vi "temperature calling.vi"() -> ()   [LabVIEW 2018]
panel:
  in  "Boolean":bool
  out "Thermometer":dbl(slide) scale=-100.0..100.0
  in  "Slide":dbl(slide) scale=0.0..100.0
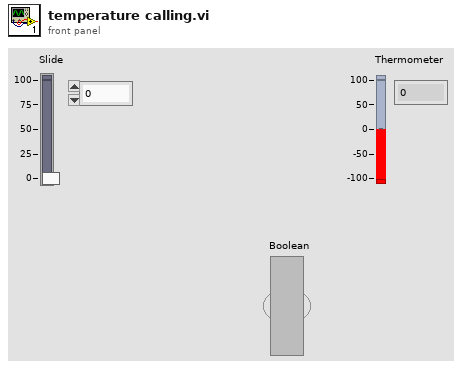
[diagram p1: front panel]
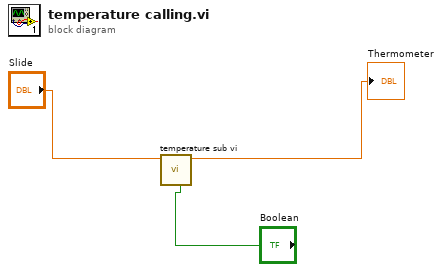
[diagram p0: block diagram]
diagram:
  n1 = call "temperature sub vi.vi"("Slide"="Slide", "Boolean"="Boolean") -> ("Numeric"=→"Thermometer":dbl)  [unwired: 7 in]
